vi "esp301 set position.vi"(7 "String":string, 8 "error in (no error)":errorcluster, 9 "Args":string[](array[string]), 10 "Seperator in":string, 11 "ESP302 in":refnum<class "ESP302.lvclass">) -> (0 "error out":errorcluster, 1 "s/mm":dbl=2.0, 2 "new commands":string, 3 "ESP302 out":refnum<class "ESP302.lvclass">, 5 "timeout":dbl)   [LabVIEW 2020, in "ESP302.lvclass"]
uses:
  ESP302.lvclass
  OnOffTypeDef.ctl
  ESP302.lvclass/ESP302.ctl
  ESP301.lvclass
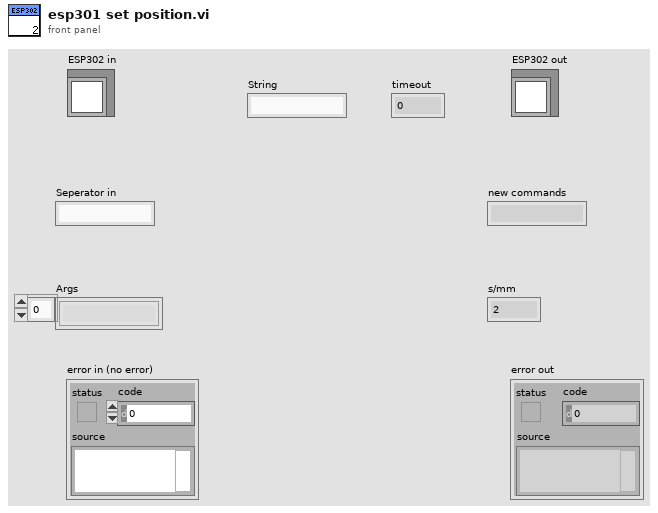
[diagram p1: front panel]
types:
  T1 = typedef "OnOffTypeDef.ctl" = enum16{"off", "on"}
  T2 = typedef "ESP301.lvclass/SettingsTypdef.ctl" = cluster{"devport":string, "Position":cluster{"Axis 1":cluster{"Value":dbl, "Min":dbl, "Max":dbl, "StepSize":dbl, "Tolerance":dbl, "ValueActual":dbl}, "Axis 2":cluster{"Value":dbl, "Min":dbl, "Max":dbl, "StepSize":dbl, "Tolerance":dbl, "ValueActual":dbl}, "Axis 3":cluster{"Value":dbl, "Min":dbl, "Max":dbl, "StepSize":dbl, "Tolerance":dbl, "ValueActual":dbl}}, "Power":cluster{"Axis 1":T1, "Axis 2":T1, "Axis 3":T1}, "Status":cluster{"Axis 1":T3, "Axis 2":T3, "Axis 3":T3}, "Backlash":cluster{"Axis 1":cluster{"Value":dbl, "Min":dbl, "Max":dbl, "StepSize":dbl, "Tolerance":dbl, "ValueActual":dbl}, "Axis 2":cluster{"Value":dbl, "Min":dbl, "Max":dbl, "StepSize":dbl, "Tolerance":dbl, "ValueActual":dbl}, "Axis 3":cluster{"Value":dbl, "Min":dbl, "Max":dbl, "StepSize":dbl, "Tolerance":dbl, "ValueActual":dbl}}, "Home":cluster{"Axis 1":cluster{"Value":dbl, "Min":dbl, "Max":dbl, "StepSize":dbl, "Tolerance":dbl, "ValueActual":dbl}, "Axis 2":cluster{"Value":dbl, "Min":dbl, "Max":dbl, "StepSize":dbl, "Tolerance":dbl, "ValueActual":dbl}, "Axis 3":cluster{"Value":dbl, "Min":dbl, "Max":dbl, "StepSize":dbl, "Tolerance":dbl, "ValueActual":dbl}}, "MoveToHardLimit":cluster{"Axis 1":T4, "Axis 2":T4, "Axis 3":T4}, "relativeMove":cluster{"Axis 1neg":T1, "Axis 2neg":T1, "Axis 3neg":T1, "Axis 1pos":T1, "Axis 2pos":T1, "Axis 3pos":T1}, "stepsize":cluster{"Value":dbl, "Min":dbl, "Max":dbl, "StepSize":dbl, "Tolerance":dbl, "ValueActual":dbl}, "automotoroff":T1, "ResetBeforeMove":T1, "Enable":cluster{"Axis 1":T1, "Axis 2":T1, "Axis 3":T1}}
  T3 = typedef "status_TypDef.ctl" = enum16{"Not referenced", "Homing", "Moving", "Ready"}
  T4 = typedef "Hardware limit.ctl" = enum16{"pos", "neg"}
  T5 = cluster{"Axis 1":cluster{"Value":dbl, "Min":dbl, "Max":dbl, "StepSize":dbl, "Tolerance":dbl, "ValueActual":dbl}, "Axis 2":cluster{"Value":dbl, "Min":dbl, "Max":dbl, "StepSize":dbl, "Tolerance":dbl, "ValueActual":dbl}, "Axis 3":cluster{"Value":dbl, "Min":dbl, "Max":dbl, "StepSize":dbl, "Tolerance":dbl, "ValueActual":dbl}}
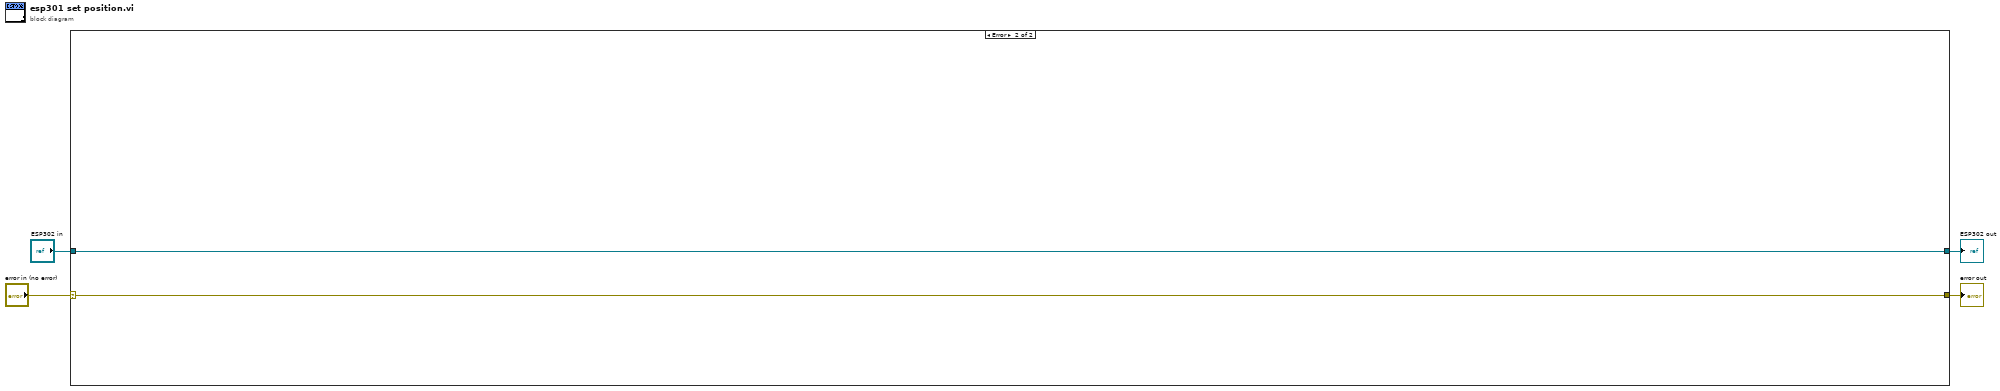
[diagram p0: block diagram]
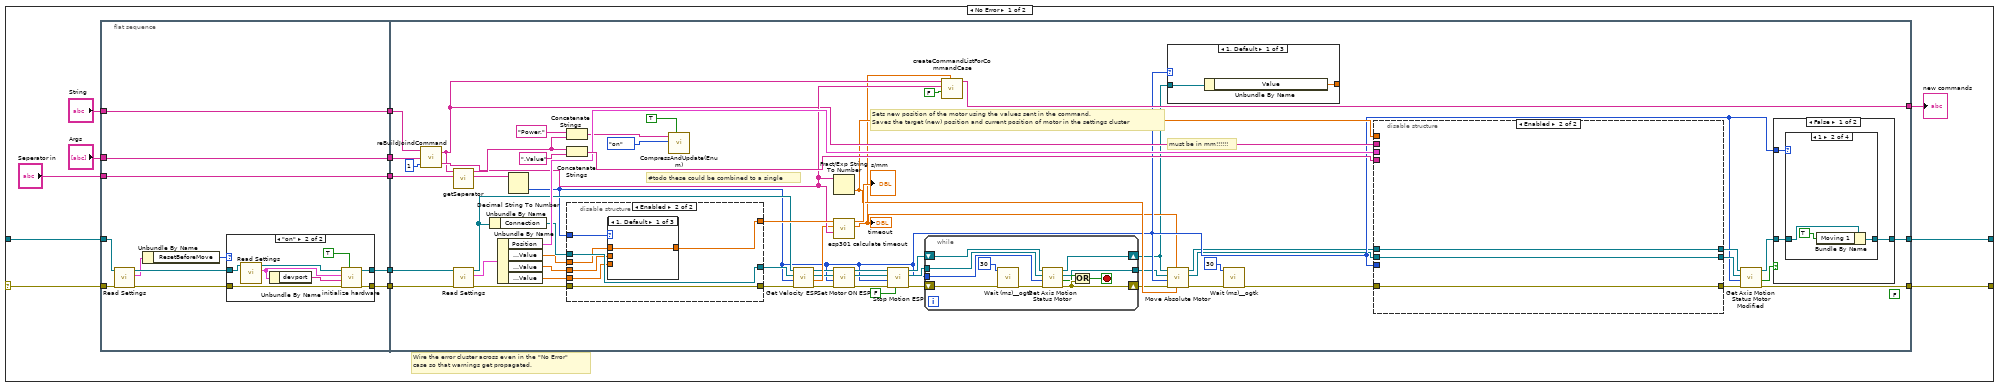
[diagram p2: hidden frame]
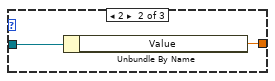
[diagram p4: hidden frame]
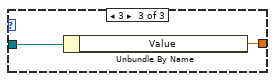
[diagram p5: hidden frame]
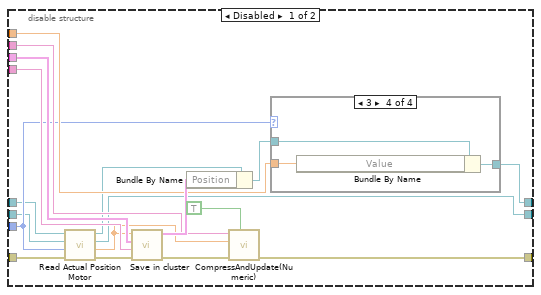
[diagram p6: hidden frame]
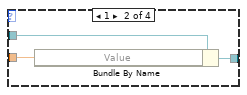
[diagram p8: hidden frame]
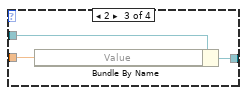
[diagram p9: hidden frame]
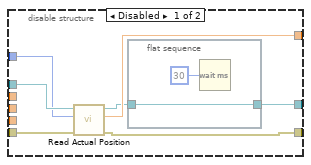
[diagram p10: hidden frame]
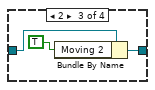
[diagram p14: hidden frame]
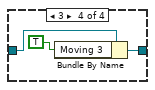
[diagram p15: hidden frame]
diagram:
  n1 = case shown="Error" "error in (no error)" {
    selector: "error in (no error)" -> [w7 w180]
    tunnel: [w5 w180] -> w3
    tunnel: [w6 w179] -> w2
    tunnel: "ESP302 in" -> [w8 w179]
    frame No Error {
      # "Wire the error cluster across even in the \"No Error\"\ncase so that warnings get propagated."
      n2 = flat-sequence {
        tunnel: w7 -> [w19]
        tunnel: w8 -> [w18]
        tunnel: "Seperator in" -> [w26]
        tunnel: "String" -> [w27]
        tunnel: "Args" -> [w28]
        tunnel: [w28] -> w17
        tunnel: [w27] -> w16
        tunnel: [w26] -> w15
        tunnel: [w25] -> w14
        tunnel: [w24] -> w13
        tunnel: [w97] -> w9
        tunnel: [w57] -> w5
        tunnel: [w89] -> w6
        tunnel: w17 -> [w95]
        tunnel: w16 -> [w94]
        tunnel: w15 -> [w93]
        tunnel: w14 -> [w52]
        tunnel: w13 -> [w50]
        frame #0 {
          n3 = call-dynamic "Read Settings.vi"("error in (no error)"=w19, "ESP301 in"=w18) -> ("error out"=w20:errorcluster, "Settings"=w21:T2, "ESP301 out"=w22:refnum<class "ESP302.lvclass">)  [unwired: 7 in]
          n4 = Unbundle By Name(w21) -> ("ResetBeforeMove"=w23:T1)
          n5 = case shown="\"on\"" w23 {
            tunnel: [w30 w38] -> w25
            tunnel: w22 -> [w30 w33]
            tunnel: w20 -> [w29 w36]
            tunnel: [w29 w35] -> w24
            frame "off", Default {
            }
            frame "on" {
              n6 = call-dynamic "Read Settings.vi"("ESP301 in"=w33) -> ("Settings"=w31:T2, "ESP301 out"=w32:refnum<class "ESP302.lvclass">)  [unwired: 8 in, 1 out]
              n7 = Unbundle By Name(w31) -> ("devport"=w37:string)
              n8 = call-dynamic "initialize hardware.vi"("Reset (False)"=TRUE, "error in (no error)"=w36, "devport"=w37, "Settings"=w31, "ESP302 in"=w32) -> ("error out"=w35:errorcluster, "ESP302 out"=w38:refnum<class "ESP302.lvclass">)  [unwired: 4 in, 1 out]
            }
          }
        }
        frame #1 {
          (unwired) FALSE
          # "#todo these could be combined to a single"
          # "must be in mm!!!!!!"
          # "Sets new position of the motor using the values sent in the command.\nSaves the target (new) position and current position of motor in the settings cluster"
          n9 = call "reBuildJoindCommand.vi"("number of group elements (0)"=1, "Args"=w95, "Command 2"=w94) -> ("Arg"=w78:string, "Command"=w77:string)
          n10 = call "getSeperator.vi"("Channel Seperator (\"\")"=w93, "Command"=w77) -> ("Channel"=w92:string, "Seperator (e.g. \"Channel1\")"=w84:string)  [unwired: 8 in]
          n11 = call-dynamic "Read Settings.vi"("error in (no error)"=w50, "ESP301 in"=w52) -> ("error out"=w51:errorcluster, "Settings"=w54:T2, "ESP301 out"=w53:refnum<class "ESP302.lvclass">)  [unwired: 7 in]
          n12 = Unbundle By Name(w53) -> ("Connection"=w80:refnum<visa-resource-name>)
          n13 = Unbundle By Name(w54) -> ("Position"=w87:T5, "Position.Axis 1.Value"=w49:dbl, "Position.Axis 2.Value"=w48:dbl, "Position.Axis 3.Value"=w47:dbl)
          n14 = Decimal String To Number(string=w92) -> (number=w46:i32)  [unwired: 2 in, 1 out]
          n15 = Concatenate Strings("Power." ("string"), w84) -> (w83:string)
          n16 = Concatenate Strings(w84, ".Value" ("string")) -> (w90:string)
          n17 = disable-structure shown="Enabled" {
            disable-tunnel: w80 -> [w141 w150]
            disable-tunnel: [w140 w148] -> w79
            disable-tunnel: [w135 w150] -> w75
            disable-tunnel: w51 -> [w139 w144]
            disable-tunnel: [w138 w144] -> w76
            disable-tunnel: w46 -> [w137 w149]
            disable-tunnel: w49 -> [_ w147]
            disable-tunnel: w48 -> [_ w146]
            disable-tunnel: w47 -> [_ w145]
            frame Disabled {
              n18 = call "Read Actual Position.vi"("error in (no error)"=w139, "Axis (1)"=w137, "VISA resource name"=w141) -> ("error out"=w138:errorcluster, "Position (units)"=w140:dbl, "VISA resource name out"=w136:refnum<visa-resource-name>)  [unwired: 2 in]
              n19 = flat-sequence {
                tunnel: w136 -> [w143]
                tunnel: [w143] -> w135
                frame #0 {
                  n20 = Wait (ms)(milliseconds to wait=u32 30) -> ()  [unwired: 1 out]
                }
              }
            }
            frame Enabled {
              n21 = case shown="1, Default" w149 {
                tunnel: [w151 w152 w153] -> w148
                tunnel: w147 -> [w151 _ _]
                tunnel: w146 -> [_ w152 _]
                tunnel: w145 -> [_ _ w153]
                frame 1, Default {
                }
                frame 2 {
                }
                frame 3 {
                }
              }
            }
          }
          n22 = call "CompressAndUpdate(Enum).vi"("force CVT update (false)"=TRUE ("force CVT update"), "enum variant"=OnOffTypeDef."on" ("Axis 1"), "command or variable name"=w83) -> ()  [unwired: 8 in, 1 out]
          n23 = call-dynamic "Get Velocity ESP.vi"("error in (no error)"=w76, "Axis (1)"=w46, "VISA resource name"=w75, "ESP302 in"=w53) -> ("error out"=w71:errorcluster, "Velocity (units/s)"=w74:dbl, "VISA resource name out"=w72:refnum<visa-resource-name>, "ESP302 out"=w73:refnum<class "ESP302.lvclass">)  [unwired: 4 in]
          n24 = Fract/Exp String To Number(string=w78) -> (number=w63:dbl)  [unwired: 3 in, 1 out]
          n25 = call "esp301 calculate timeout.vi"("Arg"=w78, "Velocity (units/s)"=w74, "Position (units)"=w79) -> ("Numeric"=w45:dbl, "Numeric 2"=→"s/mm":dbl)  [unwired: 6 in, 1 out]
          "timeout" <- w45
          n26 = call-dynamic "Set Motor ON ESP.vi"("error in (no error)"=w71, "Axis (1)"=w46, "VISA resource name"=w72, "ESP302 in"=w73) -> ("error out"=w70:errorcluster, "VISA resource name out"=w68:refnum<visa-resource-name>, "ESP302 out"=w65:refnum<class "ESP302.lvclass">)  [unwired: 5 in]
          n27 = call-dynamic "Stop Motion ESP.vi"("Stop all axes (F)"=FALSE, "error in (no error)"=w70, "Axis (1)"=w46, "VISA resource name"=w68, "ESP301 in"=w65) -> ("error out"=w66:errorcluster, "VISA resource name out"=w67:refnum<visa-resource-name>, "ESP301 out"=w64:refnum<class "ESP302.lvclass">)  [unwired: 4 in]
          n28 = while {
            tunnel: w67 -> [w177]
            tunnel: w46 -> [w173]
            tunnel: [w170] -> w44
            shift-right: [w175] -> w42
            shift-left: w66 -> [w176]
            shift-right: [w171] -> w43
            shift-left: w64 -> [w172]
            stop <- w178 stop-if-true
            n29 = call "Wait (ms)__ogtk.vi"("error in (no error)"=w176, "milliseconds to wait"=u32 30) -> ("error out"=w169:errorcluster)  [unwired: 8 in, 1 out]
            n30 = call-dynamic "Get Axis Motion Status Motor.vi"("error in (no error)"=w169, "Axis (1)"=w173, "VISA resource name"=w177, "ESP301 in"=w172) -> ("error out"=w175:errorcluster, "Motion Done"=w174:bool, "VISA resource name out"=w170:refnum<visa-resource-name>, "ESP301 out"=w171:refnum<class "ESP302.lvclass">)  [unwired: 4 in]
            n31 = Or(x=w174, y=w175) -> (x .or. y?=w178:bool)
          }
          n32 = call "createCommandListForCommandCase.vi"("timeout (optional)"=w45, "immediate Check (only once)"=FALSE, "setvalue"=w78, "command"=w77) -> ("new commands"=w97:string)  [unwired: 7 in]
          n33 = case shown="1, Default" w46 {
            tunnel: w43 -> [w99 w101 w103]
            tunnel: [w98 w100 w102] -> _
            frame 1, Default {
              n34 = Unbundle By Name(w99) -> ("Value"=w98:dbl)
            }
            frame 2 {
              n35 = Unbundle By Name(w101) -> ("Value"=w100:dbl)
            }
            frame 3 {
              n36 = Unbundle By Name(w103) -> ("Value"=w102:dbl)
            }
          }
          n37 = call-dynamic "Move Absolute Motor.vi"("Position"=w63, "timeout"=w45, "error in (no error)"=w42, "Axis"=w46, "VISA resource name in"=w44, "ESP302 in"=w43) -> ("error out"=w62:errorcluster, "VISA resource name out"=w40:refnum<visa-resource-name>, "ESP302 out"=w39:refnum<class "ESP302.lvclass">)  [unwired: 3 in]
          n38 = call "Wait (ms)__ogtk.vi"("error in (no error)"=w62, "milliseconds to wait"=u32 30) -> ("error out"=w41:errorcluster)  [unwired: 8 in, 1 out]
          n39 = disable-structure shown="Enabled" {
            disable-tunnel: [w121 w133] -> w58
            disable-tunnel: w90 -> [w120 _]
            disable-tunnel: [w104 w132] -> w56
            disable-tunnel: w40 -> [w107 w132]
            disable-tunnel: w41 -> [w111 w133]
            disable-tunnel: w87 -> [w118 _]
            disable-tunnel: [w115 w134] -> w60
            disable-tunnel: w63 -> [w114 _]
            disable-tunnel: w46 -> [w110 _]
            disable-tunnel: w77 -> [w112 _]
            disable-tunnel: w39 -> [w105 w134]
            frame Disabled {
              n40 = call-dynamic "Read Actual Position Motor.vi"("error in (no error)"=w111, "Axis (1)"=w110, "VISA resource name"=w107, "ESP301 in"=w105) -> ("error out"=w108:errorcluster, "Position (units)"=w109:dbl, "VISA resource name out"=w104:refnum<visa-resource-name>, "ESP301 out"=w106:refnum<class "ESP302.lvclass">)  [unwired: 4 in]
              n41 = call "Save in cluster.vi"("error in (no error)"=w108, "String"=w120, "Home in"=w118, "Numeric"=w109) -> ("error out"=w113:errorcluster, "Home out"=w117:T5)  [unwired: 6 in]
              n42 = Bundle By Name(cluster=w106, "Position"=w117) -> (w116:refnum<class "ESP302.lvclass">)
              n43 = call "CompressAndUpdate(Numeric).vi"("force CVT update (false)"=TRUE ("force CVT update"), "error in"=w113, "Numeric"=w109, "command or variable name"=w112) -> ("error out"=w121:errorcluster)  [unwired: 7 in]
              n44 = case shown="3" w110 {
                tunnel: w116 -> [w122 w125 w128 w131]
                tunnel: [w122 w124 w127 w130] -> w115
                tunnel: w114 -> [_ w123 w126 w129]
                frame 0, Default {
                }
                frame 1 {
                  n45 = Bundle By Name(cluster=w125, "Value"=w123) -> (w124:refnum<class "ESP302.lvclass">)
                }
                frame 2 {
                  n46 = Bundle By Name(cluster=w128, "Value"=w126) -> (w127:refnum<class "ESP302.lvclass">)
                }
                frame 3 {
                  n47 = Bundle By Name(cluster=w131, "Value"=w129) -> (w130:refnum<class "ESP302.lvclass">)
                }
              }
            }
            frame Enabled {
            }
          }
          n48 = call-dynamic "Get Axis Motion Status Motor Modified.vi"("error in (no error)"=w58, "Axis (1)"=w46, "VISA resource name"=w56, "ESP302 in"=w60) -> ("error out"=w57:errorcluster, "Motion Done"=w55:bool, "ESP302 out"=w59:refnum<class "ESP302.lvclass">)  [unwired: 4 in, 1 out]
          n49 = case shown="False" w55 {
            tunnel: w46 -> [w156 _]
            tunnel: w59 -> [w155 w167]
            tunnel: [w154 w167] -> w89
            frame False {
              n50 = case shown="1" w156 {
                tunnel: w155 -> [w157 w160 w163 w166]
                tunnel: [w157 w159 w162 w165] -> w154
                frame 0, Default {
                }
                frame 1 {
                  n51 = Bundle By Name(cluster=w160, "Moving 1"=TRUE) -> (w159:refnum<class "ESP302.lvclass">)
                }
                frame 2 {
                  n52 = Bundle By Name(cluster=w163, "Moving 2"=TRUE) -> (w162:refnum<class "ESP302.lvclass">)
                }
                frame 3 {
                  n53 = Bundle By Name(cluster=w166, "Moving 3"=TRUE) -> (w165:refnum<class "ESP302.lvclass">)
                }
              }
            }
            frame True {
            }
          }
        }
      }
      "new commands" <- w9
    }
    frame Error {
    }
  }
  "error out" <- w3
  "ESP302 out" <- w2
